vi "Position Panel (top left).vi"(0 "reference":refnum<vi>, 5 "Top":i16, 7 "Left":i16, 9 "Height":i16, 11 "error in (no error)":errorcluster) -> (4 "reference out":refnum<vi>, 8 "Width out":i16, 10 "Height out":i16, 15 "error out":errorcluster)   [LabVIEW 2015]
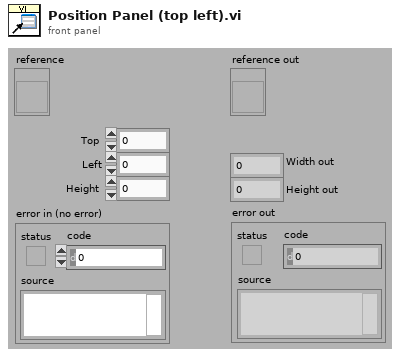
[diagram p1: front panel]
types:
  T1 = typedef "LVRectTypeDef.ctl" = cluster{"Left":i16, "Top":i16, "Right":i16, "Bottom":i16}
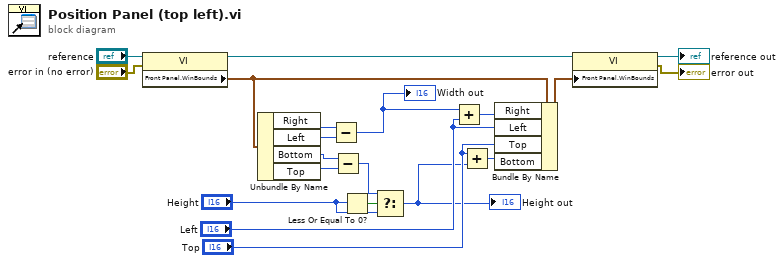
[diagram p0: block diagram]
diagram:
  n1 = property class="VI"(reference="reference", error in="error in (no error)") -> (reference out=w1:refnum<vi>, "Front Panel.WinBounds"=w15:T1)  [unwired: 1 out]
  n2 = Unbundle By Name(w15) -> ("Right"=w13:i16, "Left"=w14:i16, "Bottom"=w12:i16, "Top"=w11:i16)
  n3 = Subtract(x=w13, y=w14) -> (x-y=w3:i16)
  "Width out" <- w3
  n4 = Subtract(x=w12, y=w11) -> (x-y=w4:i16)
  n5 = Less Or Equal To 0?(x="Height") -> (x <= 0?=w6:bool)
  n6 = Select(t=w4, s=w6, f="Height") -> (s? t:f=w2:i16)
  "Height out" <- w2
  n7 = Add(x=w3, y="Left") -> (x+y=w8:i16)
  n8 = Add(x="Top", y=w2) -> (x+y=w10:i16)
  n9 = Bundle By Name(cluster=w15, "Right"=w8, "Left"="Left", "Top"="Top", "Bottom"=w10) -> (w18:T1)
  n10 = property class="VI"(reference=w1, "Front Panel.WinBounds"=w18) -> (reference out=→"reference out":refnum<vi>, error out=→"error out":errorcluster)  [unwired: 1 in]
